vi "6. CoffeeMaker Data Management.vi"() -> ()   [LabVIEW 2018]
doc: "Coffee Machine Version 1.0: first examples for data management in state machines"
uses:
  Controls/States.ctl
  <vilib>/Utility/miscctls.llb/LVMinMaxIncTypeDef.ctl
  <vilib>/Utility/file.llb/Read Delimited Spreadsheet (string).vi
panel:
  out "s? t:f":enum16{"next state", "current state"}(ring)
  out "error out":errorcluster
  in  "error in (no error)":errorcluster
  in  "Power Switch":bool
  in  "Simulation":cluster{"Water":dbl, "Coffee":dbl, "Milk":dbl} caption="Wasser" {"Milk" scale=0.0..100.0; "Water" scale=0.0..100.0; "Coffee" scale=0.0..100.0}
  out "Display":T1 {"Coffee" scale=0.0..80.0; "Brewing Chamber" scale=0.0..80.0}
  in  "Coffee Selection":T2 {"Type" min=0 max=0 step=1 scale=0.0..2.0}
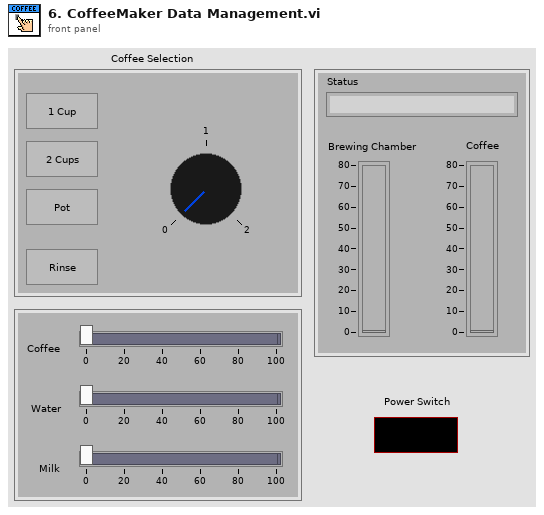
[diagram p1: front panel]
types:
  T1 = cluster{"Brewing Chamber":dbl, "Coffee":dbl, "Status":string}
  T2 = cluster{"1 Cup":bool, "2 Cups":bool, "Pot":bool, "Rinse":bool, "Type":i8}
  T3 = cluster{"Status":refnum<vi>, "Brewing Chamber":refnum<vi>, "Coffee":refnum<vi>, "Power Switch":refnum<vi>}
  T4 = typedef "States.ctl" = enum16{"Initialize", "Set Language", "Wait for Power On", "Heat up", "Check and Wait for Water", "Rinsing", "Check Resources", "User Input", "Grinding", "Boiling", "Pouring", "Rinse before Stop", "Write Data", "Stop"}
  T5 = enum8{"Enabled", "Disabled", "Disabled and Grayed Out"}
  T6 = typedef "LVMinMaxIncTypeDef.ctl" = cluster{"Minimum":dbl, "Maximum":dbl, "Increment":dbl}
  T7 = cluster{"Coffee":refnum<vi>, "Water":refnum<vi>, "Milk":refnum<vi>}
  T8 = cluster{"Coffee Selection":refnum<vi>, "1 Cup":refnum<vi>, "2 Cups":refnum<vi>, "Pot":refnum<vi>, "Rinse":refnum<vi>, "Type":refnum<vi>}
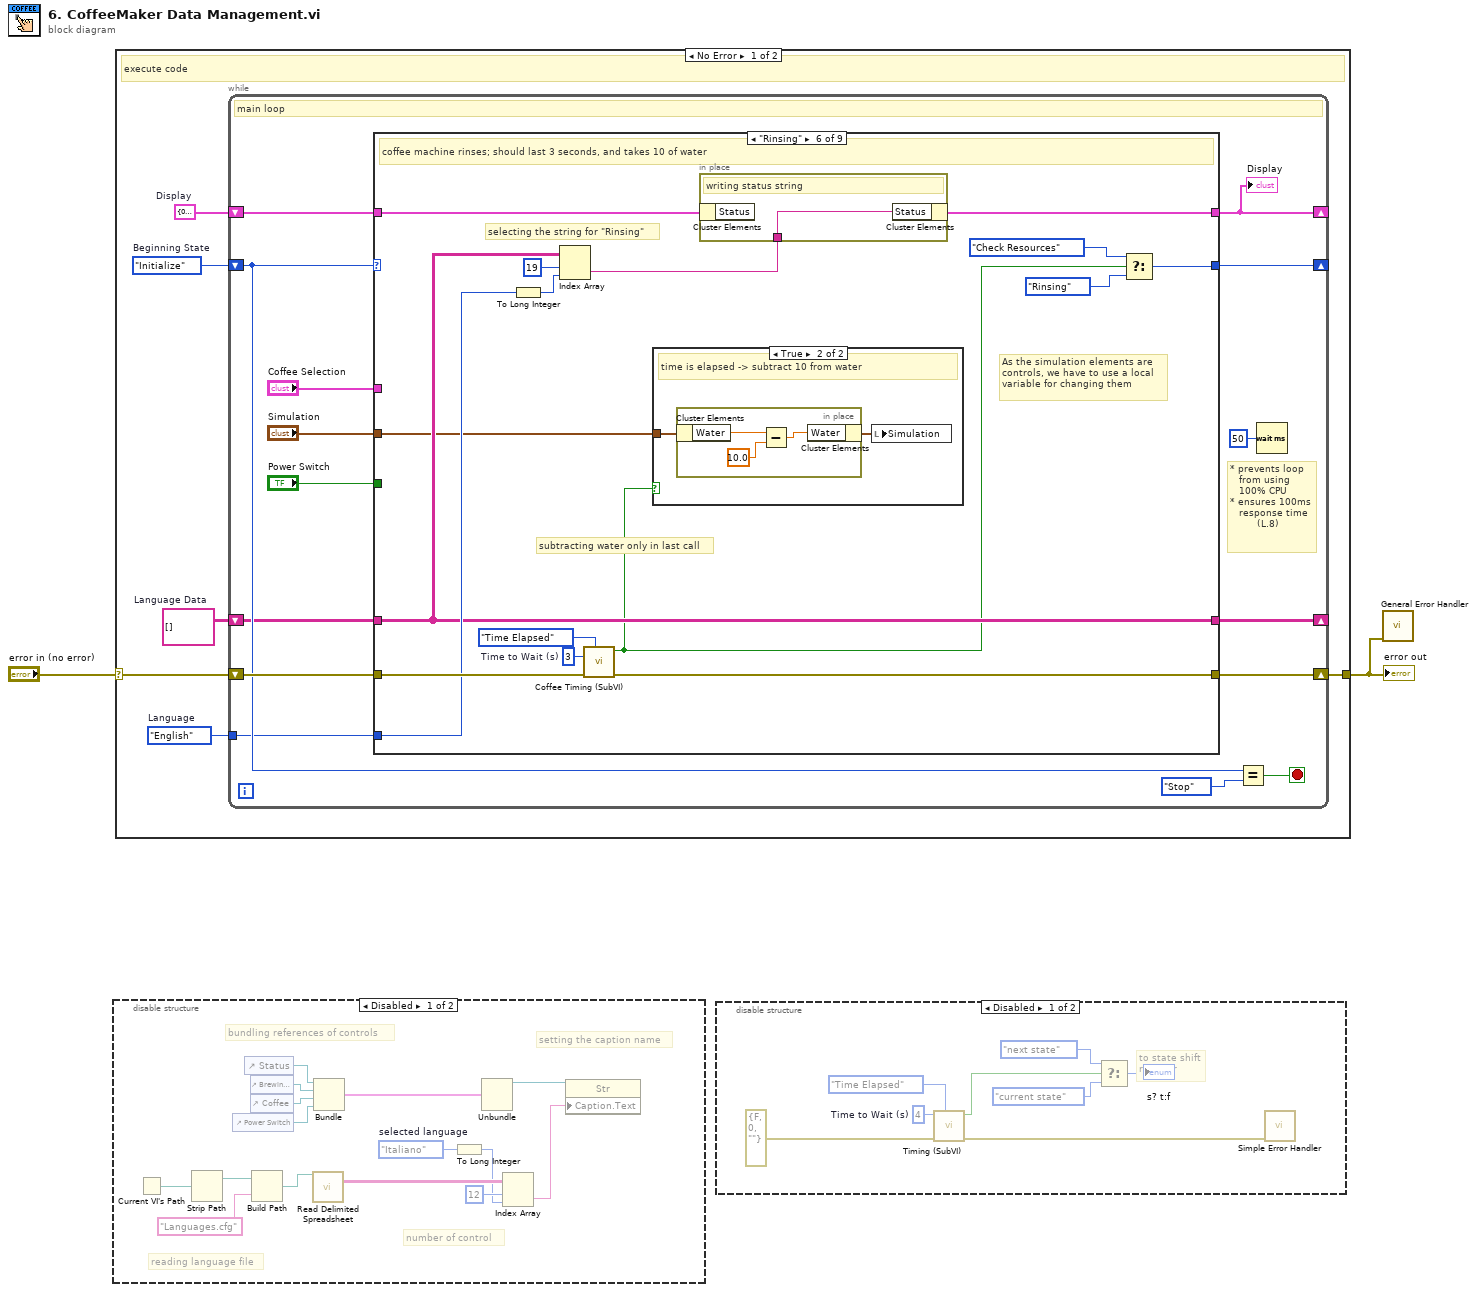
[diagram p0: block diagram]
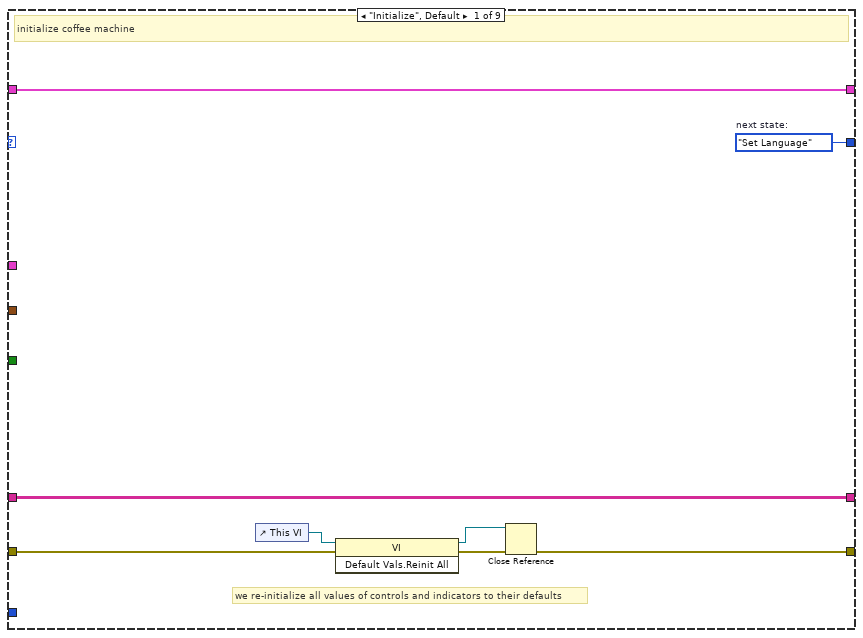
[diagram p4: hidden frame]
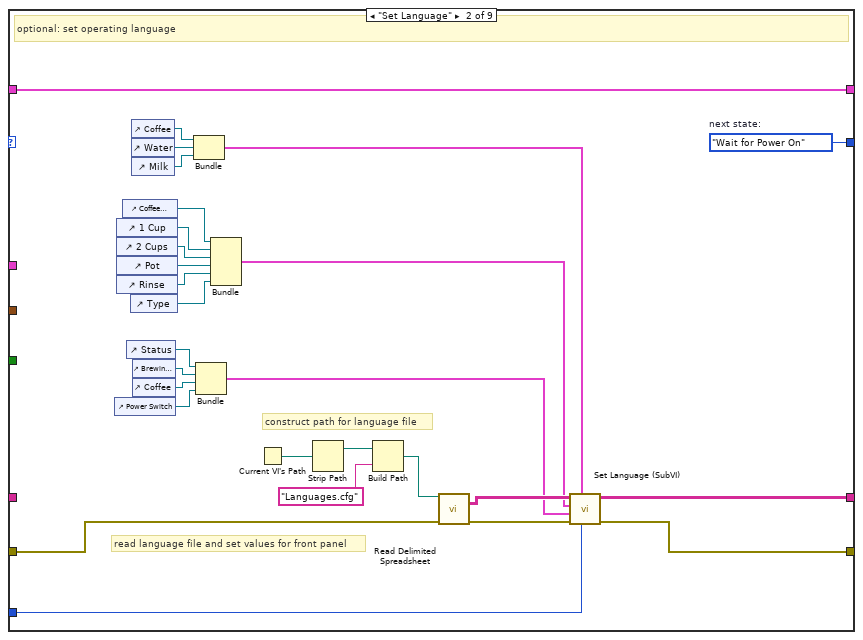
[diagram p5: hidden frame]
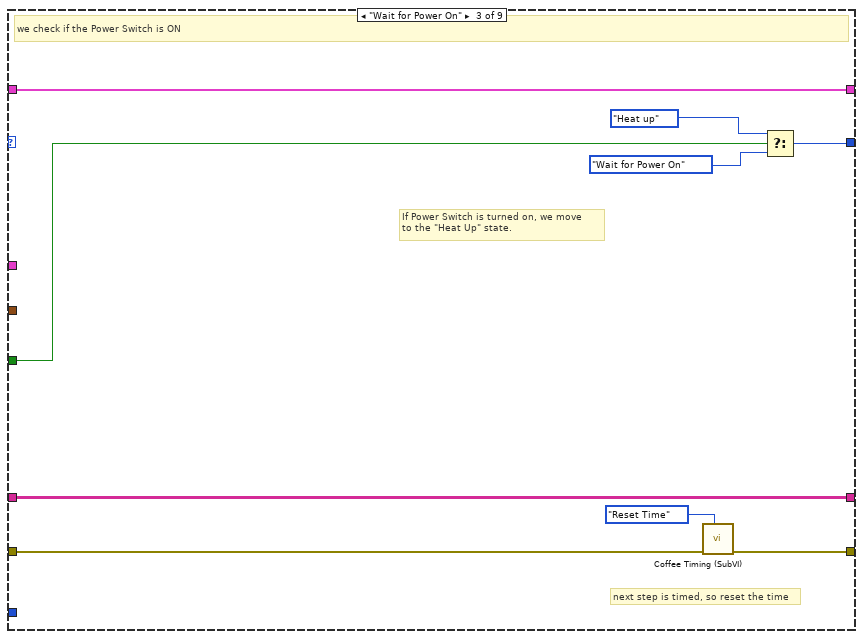
[diagram p6: hidden frame]
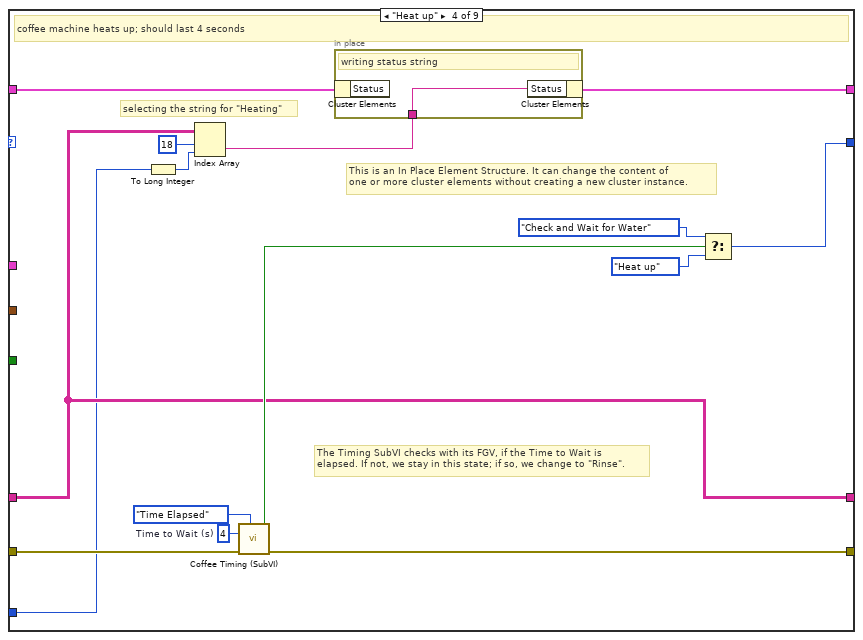
[diagram p7: hidden frame]
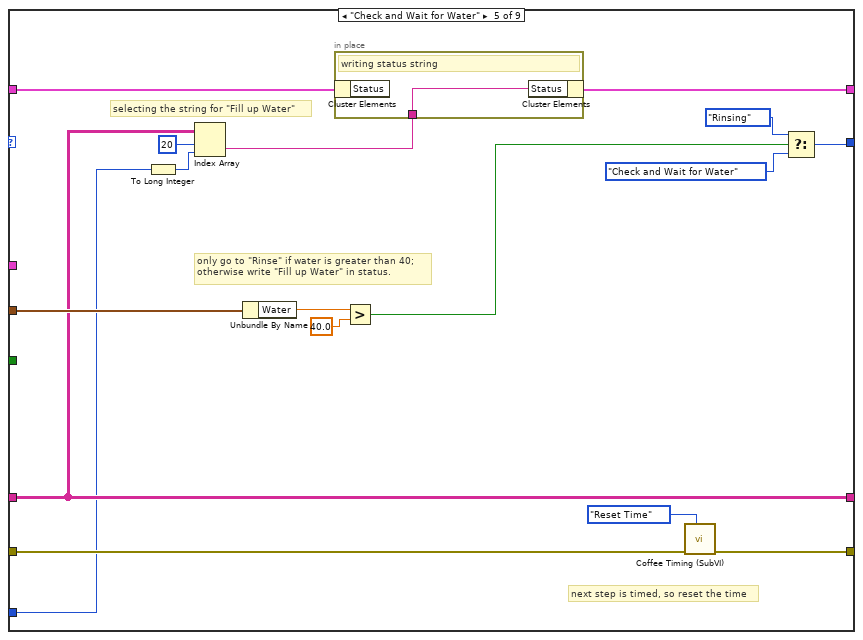
[diagram p8: hidden frame]
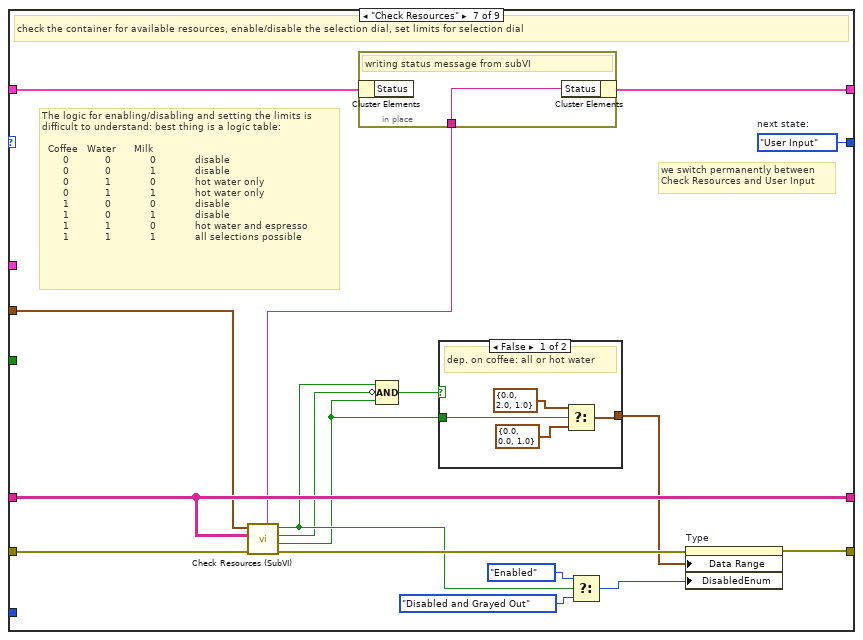
[diagram p10: hidden frame]
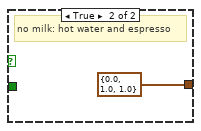
[diagram p11: hidden frame]
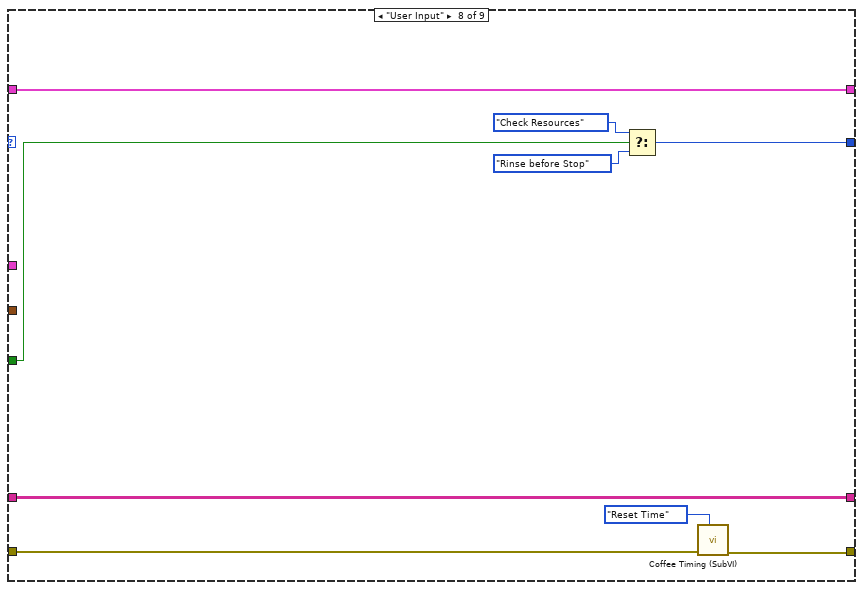
[diagram p12: hidden frame]
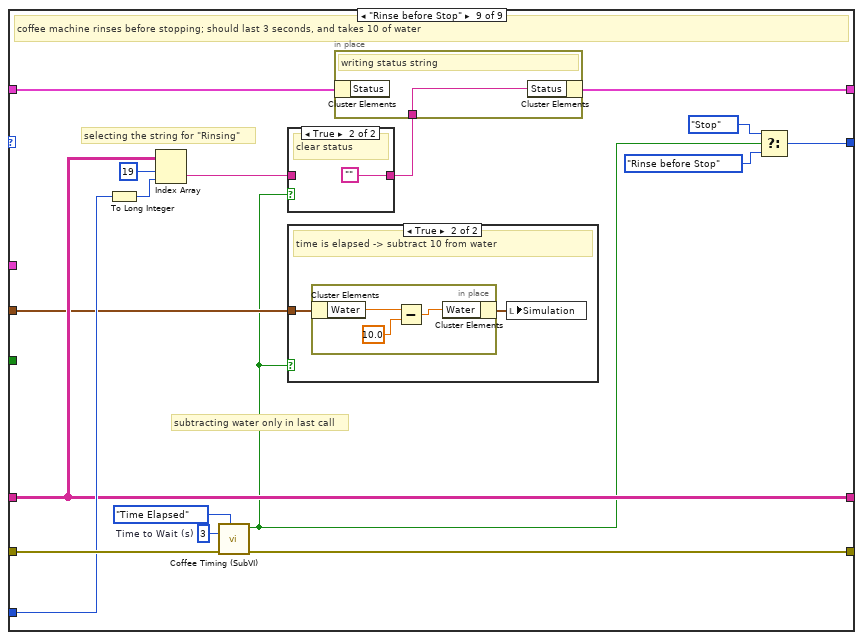
[diagram p13: hidden frame]
diagram:
  n1 = disable-structure shown="Disabled" {
    frame Disabled {
      w5 = enum16{"English", "Deutsch", "Italiano"}."Italiano"  # selected language
      # "setting the caption name"
      # "number of control"
      # "reading language file"
      # "bundling references of controls"
      n2 = Current VI's Path() -> (path=w11:path)
      n3 = Strip Path(path=w11) -> (stripped path=w10:path)  [unwired: 1 out]
      n4 = control-ref of="Power Switch"() -> (w17:refnum<vi>)
      n5 = control-ref of="Status"() -> (w14:refnum<vi>)
      n6 = control-ref of="Brewing Chamber"() -> (w15:refnum<vi>)
      n7 = control-ref of="Coffee"() -> (w16:refnum<vi>)
      n8 = Build Path(base path=w10, name or relative path="Languages.cfg") -> (appended path=w8:path)
      n9 = call-poly <vilib>:"Read Delimited Spreadsheet.vi"("file path (dialog if empty)"=w8) -> ("all rows"=w7:string[][])  [unwired: 9 in, 5 out]
      n10 = Bundle("Status"=w14, "Brewing Chamber"=w15, "Coffee"=w16, "Power Switch"=w17) -> (w13:T3)  [unwired: 1 in]
      n11 = To Long Integer(number=w5) -> (32bit integer=w4:i32)
      n12 = Unbundle(w13) -> ("Status"=w12:refnum<vi>)  [unwired: 3 out]
      n13 = Index Array(array=w7, index (row)=12, index (col)=w4) -> (element=w3:string)
      n14 = property class="Str"(reference=w12, "Caption.Text"=w3) -> ()  [unwired: 1 in, 2 out]
    }
    frame Enabled {
    }
  }
  n15 = case shown="No Error" "error in (no error)" {
    selector: "error in (no error)" -> [w22 w197]
    tunnel: [w23 w197] -> w1
    frame No Error {
      w18 = enum16{"English", "Deutsch", "Italiano"}."English"  # Language
      w19 = string[][] []  # Language Data
      w20 = T1 {"Brewing Chamber"=0.0, "Coffee"=0.0, "Status"=""}  # Display
      w21 = States."Initialize"  # Beginning State
      # "execute code"
      n16 = while {
        shift-right: [w35] -> _
        shift-left: w21 -> [w34]
        shift-right: [w28] -> _
        shift-left: w19 -> [w26]
        shift-right: [w27] -> _
        shift-left: w20 -> [w31]
        shift-right: [w38] -> w23
        shift-left: w22 -> [w37]
        tunnel: w18 -> [w24]
        stop <- w32 stop-if-true
        # "* prevents loop\n   from using\n   100% CPU\n* ensures 100ms\n   response time\n         (L.8)"
        # "main loop"
        n17 = case shown="\"Rinsing\"" w34 {
          tunnel: [w40 w67 w78 w97 w107 w132 w146 w168 w187] -> w38
          tunnel: w37 -> [w45 w68 w79 w98 w108 w133 w156 w169 w188]
          tunnel: "Power Switch" -> [_ _ w83 _ _ _ _ w166 _]
          tunnel: [w42 w61 w82 w94 w114 w129 w150 w164 w184] -> w35
          tunnel: [w41 w60 w76 w89 w100 w125 w151 w170 w181] -> w27
          tunnel: w31 -> [w41 w60 w76 w90 w106 w126 w153 w170 w182]
          tunnel: "Coffee Selection" -> [_ _ _ _ _ _ _ _ _]
          tunnel: "Simulation" -> [_ _ _ _ w113 w118 w154 _ w176]
          tunnel: [w39 w66 w75 w88 w103 w121 w155 w171 w177] -> w28
          tunnel: w26 -> [w39 _ w75 w88 w103 w121 w155 w171 w177]
          tunnel: w24 -> [_ w47 _ w85 w102 w122 _ _ w178]
          frame "Initialize", Default {
            w42 = States."Set Language"  # next state:
            # "we re-initialize all values of controls and indicators to their defaults"
            # "initialize coffee machine"
            n18 = control-ref of="This VI"() -> (w46:refnum<vi>)
            n19 = invoke class="VI" method="Default Vals.Reinit All"(reference=w46, error in=w45) -> (reference out=w44:refnum<vi>, error out=w43:errorcluster)  [unwired: 1 in, 1 out]
            n20 = Close Reference(reference=w44, error in (no error)=w43) -> (error out=w40:errorcluster)
          }
          frame "Set Language" {
            w61 = States."Wait for Power On"  # next state:
            # "construct path for language file"
            # "read language file and set values for front panel"
            # "optional: set operating language"
            n21 = control-ref of="Power Switch"() -> (w50:refnum<vi>)
            n22 = control-ref of="1 Cup"() -> (w58:refnum<vi>)
            n23 = control-ref of="2 Cups"() -> (w57:refnum<vi>)
            n24 = control-ref of="Pot"() -> (w56:refnum<vi>)
            n25 = control-ref of="Rinse"() -> (w55:refnum<vi>)
            n26 = control-ref of="Coffee Selection"() -> (w59:refnum<vi>)
            n27 = control-ref of="Status"() -> (w53:refnum<vi>)
            n28 = control-ref of="Type"() -> (w54:refnum<vi>)
            n29 = control-ref of="Coffee"() -> (w64:refnum<vi>)
            n30 = control-ref of="Water"() -> (w63:refnum<vi>)
            n31 = control-ref of="Milk"() -> (w62:refnum<vi>)
            n32 = control-ref of="Brewing Chamber"() -> (w52:refnum<vi>)
            n33 = control-ref of="Coffee"() -> (w51:refnum<vi>)
            n34 = Bundle("Coffee"=w64, "Water"=w63, "Milk"=w62) -> (w65:T7)  [unwired: 1 in]
            n35 = Bundle("Status"=w53, "Brewing Chamber"=w52, "Coffee"=w51, "Power Switch"=w50) -> (w48:T3)  [unwired: 1 in]
            n36 = Bundle("Coffee Selection"=w59, "1 Cup"=w58, "2 Cups"=w57, "Pot"=w56, "Rinse"=w55, "Type"=w54) -> (w49:T8)  [unwired: 1 in]
            n37 = Current VI's Path() -> (path=w69:path)
            n38 = Strip Path(path=w69) -> (stripped path=w70:path)  [unwired: 1 out]
            n39 = Build Path(base path=w70, name or relative path="Languages.cfg") -> (appended path=w72:path)
            n40 = call-poly <vilib>:"Read Delimited Spreadsheet.vi"("file path (dialog if empty)"=w72, "error in (no error)"=w68) -> ("all rows"=w74:string[][], "error out"=w73:errorcluster)  [unwired: 8 in, 4 out]
            n41 = call "Set Language (SubVI).vi"("Language (English)"=w47, "Simulation \nReferences"=w65, "error in (no error)"=w73, "Status\nReferences"=w48, "Selection \nReferences"=w49, "Language Data"=w74) -> ("error out"=w67:errorcluster, "Language Data Out"=w66:string[][])  [unwired: 4 in]
          }
          frame "Wait for Power On" {
            # "next step is timed, so reset the time"
            # "If Power Switch is turned on, we move\nto the \"Heat Up\" state."
            # "we check if the Power Switch is ON"
            n42 = call "Coffee Timing (SubVI).vi"("Function"=enum16{"Reset Time", "Time Elapsed"}."Reset Time", "error in (no error)"=w79) -> ("error out"=w78:errorcluster)  [unwired: 7 in, 2 out]
            n43 = Select(t=States."Heat up" ("Beginning State"), s=w83, f=States."Wait for Power On") -> (s? t:f=w82:T4)
          }
          frame "Heat up" {
            w95 = 4  # Time to Wait (s)
            # "selecting the string for \"Heating\""
            # "This is an In Place Element Structure. It can change the content of\none or more cluster elements without creating a new cluster instance."
            # "The Timing SubVI checks with its FGV, if the Time to Wait is\nelapsed. If not, we stay in this state; if so, we change to \"Rinse\"."
            # "coffee machine heats up; should last 4 seconds"
            n44 = To Long Integer(number=w85) -> (32bit integer=w86:i32)
            n45 = Index Array "Index Array"(array=w88, index (row)=18, index (col)=w86) -> (element=w84:string)
            n46 = call "Coffee Timing (SubVI).vi"("Function"=enum16{"Reset Time", "Time Elapsed"}."Time Elapsed", "error in (no error)"=w98, "Time to Wait (s)"=w95) -> ("error out"=w97:errorcluster, "Time elapsed ?"=w91:bool)  [unwired: 6 in, 1 out]
            n47 = in-place {
              in-place-border: w84 -> [w99]
              # "writing status string"
              n48 = in-place-cluster #1(w90) -> ()  [unwired: 1 out]
              n49 = in-place-cluster #1("Status"=w99) -> (w89:T1)
            }
            n50 = Select(t=States."Check and Wait for Water" ("Beginning State"), s=w91, f=States."Heat up" ("Beginning State")) -> (s? t:f=w94:T4)
          }
          frame "Check and Wait for Water" {
            # "next step is timed, so reset the time"
            # "only go to \"Rinse\" if water is greater than 40;\notherwise write \"Fill up Water\" in status."
            # "selecting the string for \"Fill up Water\""
            n51 = To Long Integer(number=w102) -> (32bit integer=w104:i32)
            n52 = Index Array "Index Array"(array=w103, index (row)=20, index (col)=w104) -> (element=w101:string)
            n53 = Unbundle By Name(w113) -> ("Water"=w112:dbl)
            n54 = in-place {
              in-place-border: w101 -> [w117]
              # "writing status string"
              n55 = in-place-cluster #2(w106) -> ()  [unwired: 1 out]
              n56 = in-place-cluster #2("Status"=w117) -> (w100:T1)
            }
            n57 = Greater?(x=w112, y=40.0) -> (0:w110:bool)
            n58 = call "Coffee Timing (SubVI).vi"("Function"=enum16{"Reset Time", "Time Elapsed"}."Reset Time", "error in (no error)"=w108) -> ("error out"=w107:errorcluster)  [unwired: 7 in, 2 out]
            n59 = Select(t=States."Rinsing" ("f"), s=w110, f=States."Check and Wait for Water") -> (s? t:f=w114:T4)
          }
          frame "Rinsing" {
            w130 = 3  # Time to Wait (s)
            # "subtracting water only in last call"
            # "As the simulation elements are\ncontrols, we have to use a local\nvariable for changing them"
            # "selecting the string for \"Rinsing\""
            # "coffee machine rinses; should last 3 seconds, and takes 10 of water"
            n60 = To Long Integer(number=w122) -> (32bit integer=w123:i32)
            n61 = Index Array "Index Array"(array=w121, index (row)=19, index (col)=w123) -> (element=w120:string)
            n62 = call "Coffee Timing (SubVI).vi"("Function"=enum16{"Reset Time", "Time Elapsed"}."Time Elapsed", "error in (no error)"=w133, "Time to Wait (s)"=w130) -> ("error out"=w132:errorcluster, "Time elapsed ?"=w119:bool)  [unwired: 6 in, 1 out]
            n63 = case shown="True" w119 {
              tunnel: w118 -> [_ w135]
              frame False {
                # "time is running ..."
              }
              frame True {
                # "time is elapsed -> subtract 10 from water"
                n64 = in-place {
                  n65 = in-place-cluster #3(w135) -> ("Water"=w138:dbl)
                  n66 = Subtract(x=w138, y=10.0) -> (x-y=w136:dbl)
                  n67 = in-place-cluster #3("Water"=w136) -> (w134:cluster{"Water":dbl, "Coffee":dbl, "Milk":dbl})
                }
                n68 = local write "Simulation"(w134) -> ()
              }
            }
            n69 = in-place {
              in-place-border: w120 -> [w139]
              # "writing status string"
              n70 = in-place-cluster #4(w126) -> ()  [unwired: 1 out]
              n71 = in-place-cluster #4("Status"=w139) -> (w125:T1)
            }
            n72 = Select(t=States."Check Resources" ("Beginning State"), s=w119, f=States."Rinsing" ("Beginning State")) -> (s? t:f=w129:T4)
          }
          frame "Check Resources" {
            w150 = States."User Input"  # next state:
            # "The logic for enabling/disabling and setting the limits is \ndifficult to understand: best thing is a logic table:\n\n  Coffee   Water      Milk\n       0            0             0             disable\n       0            0             1             disable\n       0            1             0             hot water only\n       0            1             1             hot water only\n       1            0             0             disable\n       1            0             1             disable\n       1            1             0             hot water and espresso\n       1            1             1             all selections possible"
            # "we switch permanently between \nCheck Resources and User Input"
            # "check the container for available resources, enable/disable the selection dial, set limits for selection dial"
            n73 = call "Check Resources (SubVI).vi"("error in (no error)"=w156, "Language Data"=w155, "Simulation"=w154) -> ("error out"=w147:errorcluster, "Coffee ok?"=w141:bool, "Milk ok?"=w143:bool, "Water ok?"=w144:bool, "Status Message"=w152:string)  [unwired: 4 in]
            n74 = in-place {
              in-place-border: w152 -> [w162]
              # "writing status message from subVI"
              n75 = in-place-cluster #5(w153) -> ()  [unwired: 1 out]
              n76 = in-place-cluster #5("Status"=w162) -> (w151:T1)
            }
            n77 = Compound Arithmetic op=AND(w144, invert w143, w141) -> (w142:bool)
            n78 = case shown="False" w142 {
              tunnel: w141 -> [w158 _]
              tunnel: [w157 T6 {"Minimum"=0.0, "Maximum"=1.0, "Increment"=1.0} ("Data Entry Limits")] -> w140
              frame False {
                # "dep. on coffee: all or hot water"
                n79 = Select(t=T6 {"Minimum"=0.0, "Maximum"=2.0, "Increment"=1.0} ("Data Entry Limits"), s=w158, f=T6 {"Minimum"=0.0, "Maximum"=0.0, "Increment"=1.0} ("Data Entry Limits")) -> (s? t:f=w157:T6)
              }
              frame True {
                # "no milk: hot water and espresso"
              }
            }
            n80 = Select(t=T5."Enabled" ("Disabled"), s=w144, f=T5."Disabled and Grayed Out" ("Disabled")) -> (s? t:f=w145:T5)
            n81 = property on="Type" class="Knob (strict)"(error in=w147, "Data Range"=w140, "DisabledEnum"=w145) -> (error out=w146:errorcluster)  [unwired: 1 in, 1 out]
          }
          frame "User Input" {
            n82 = Select(t=States."Check Resources" ("Beginning State"), s=w166, f=States."Rinse before Stop") -> (s? t:f=w164:T4)
            n83 = call "Coffee Timing (SubVI).vi"("Function"=enum16{"Reset Time", "Time Elapsed"}."Reset Time", "error in (no error)"=w169) -> ("error out"=w168:errorcluster)  [unwired: 7 in, 2 out]
          }
          frame "Rinse before Stop" {
            w185 = 3  # Time to Wait (s)
            # "subtracting water only in last call"
            # "selecting the string for \"Rinsing\""
            # "coffee machine rinses before stopping; should last 3 seconds, and takes 10 of water"
            n84 = To Long Integer(number=w178) -> (32bit integer=w179:i32)
            n85 = Index Array "Index Array"(array=w177, index (row)=19, index (col)=w179) -> (element=w172:string)
            n86 = call "Coffee Timing (SubVI).vi"("Function"=enum16{"Reset Time", "Time Elapsed"}."Time Elapsed", "error in (no error)"=w188, "Time to Wait (s)"=w185) -> ("error out"=w187:errorcluster, "Time elapsed ?"=w174:bool)  [unwired: 6 in, 1 out]
            n87 = case shown="True" w174 {
              tunnel: [w189 ""] -> w173
              tunnel: w172 -> [w189 _]
              frame False {
                # "write status"
              }
              frame True {
                # "clear status"
              }
            }
            n88 = case shown="True" w174 {
              tunnel: w176 -> [_ w192]
              frame False {
                # "time is running ..."
              }
              frame True {
                # "time is elapsed -> subtract 10 from water"
                n89 = in-place {
                  n90 = in-place-cluster #6(w192) -> ("Water"=w195:dbl)
                  n91 = Subtract(x=w195, y=10.0) -> (x-y=w193:dbl)
                  n92 = in-place-cluster #6("Water"=w193) -> (w191:cluster{"Water":dbl, "Coffee":dbl, "Milk":dbl})
                }
                n93 = local write "Simulation"(w191) -> ()
              }
            }
            n94 = in-place {
              in-place-border: w173 -> [w196]
              # "writing status string"
              n95 = in-place-cluster #7(w182) -> ()  [unwired: 1 out]
              n96 = in-place-cluster #7("Status"=w196) -> (w181:T1)
            }
            n97 = Select(t=States."Stop" ("Beginning State"), s=w174, f=States."Rinse before Stop") -> (s? t:f=w184:T4)
          }
        }
        "Display" <- w27
        n98 = Equal?(x=w34, y=States."Stop") -> (x = y?=w32:bool)
        n99 = Wait (ms)(milliseconds to wait=u32 50) -> ()  [unwired: 1 out]
      }
    }
    frame Error {
      # "do nothing"
    }
  }
  "error out" <- w1
  n100 = disable-structure shown="Disabled" {
    frame Disabled {
      w204 = 4  # Time to Wait (s)
      # "to state shift\nregister"
      n101 = call "Timing (SubVI).vi"("Function"=enum16{"Reset Time", "Time Elapsed"}."Time Elapsed", "error in (no error)"=errorcluster {"status"=FALSE, "code"=0, "source"=""}, "Time to Wait (s)"=w204) -> ("error out"=w202:errorcluster, "Time elapsed ?"=w201:bool)  [unwired: 6 in, 1 out]
      n102 = Select(t=enum16{"next state", "current state"}."next state", s=w201, f=enum16{"next state", "current state"}."current state") -> (s? t:f=→"s? t:f":enum16{"next state", "current state"})
      n103 = call <vilib>:"Simple Error Handler.vi"("error in (no error)"=w202) -> ()  [unwired: 4 in, 5 out]
    }
    frame Enabled {
    }
  }
  n104 = call <vilib>:"General Error Handler.vi"("error in (no error)"=w1) -> ()  [unwired: 10 in, 5 out]
